vi "Type Conversion.To Double (1D I32).vi"(3 "values in":i32[](array[numeric])) -> (1 "values out":dbl[](array[numeric]))   [LabVIEW 2016, in "VeriStand Data.lvlib"]
doc: "Converts the provided values to double floats, preserving the numerical value of the data."
uses:
  VeriStand Data.lvlib
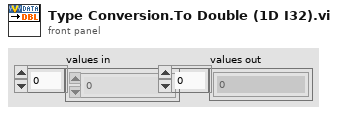
[diagram p1: front panel]
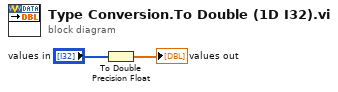
[diagram p0: block diagram]
diagram:
  n1 = To Double Precision Float(number="values in") -> (double precision float=→"values out":dbl[])
